vi "Create Occurance.vi"(8 "error in (no error)":errorcluster) -> (0 "error out":errorcluster, 2 "Occurrence User Event":refnum<user-event>, 3 "Occurrence":refnum<event-registration>)   [LabVIEW 2024, in "grpc-lvsupport.lvlib"]
uses:
  grpc-lvsupport.lvlib
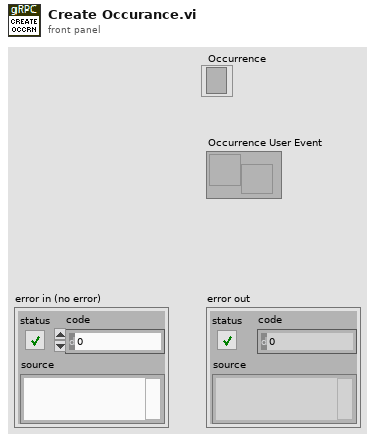
[diagram p1: front panel]
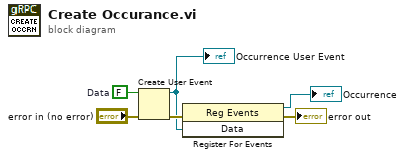
[diagram p0: block diagram]
diagram:
  w4 = FALSE  # Data
  n1 = Create User Event(user event datatype=w4, error in="error in (no error)") -> (user event=w1:refnum<user-event>, error out=w5:errorcluster)
  "Occurrence User Event" <- w1
  n2 = register-events(error in=w5, w1) -> (reference out=→"Occurrence":refnum<event-registration>, error out=→"error out":errorcluster)  [unwired: 1 in]
